vi "ADC Data capture and Process Original - Copy (2).vi"(0 "ADC Output Read Method":T2(ring)=enum."Read .dat file", 1 "Select the Tab to project":T1(ring)=enum."ADC Sine", 2 "ADC Input":enum16{"Sine Wave", "Ramp / Triangle"}(ring), 3 "No.of samples(SNR)":i32=4096, 4 "Resolution":i32=12, 5 "active edge":i32(ring)=10280, 6 "Inputs for Dyanmic para":T9={"Fundamental Frequency"=100000.0, "Sampling Frequncy"=3999610.0, "No of Harmonics"=9, "Window"=enum."7 Term B-Harris", "Blackman (fundamental power) bins)"=1.0}, 7 "Samples per Channel":i32=4096 caption="No.of Samples(capture)", 8 "Oversampling":bool, 9 "Oversampling ratio":i32, 10 "Drop LSB":bool, 11 "Save data":T15, 12 "Waveform":i64[](array[numeric]), 13 "Path to Read":path=path "C/Users/a0230227/Desktop/save.dat", 14 "Start & Stop Bit":cluster{"Start":i32, "Stop":i32}={"Start"=40, "Stop"=4055}, 15 "length":i32=4096, 17 "Set_Freq":dbl=100017.0, 24 "path to save":T14={"Path to Save plot"=path "D/Tenor_176P/DYN_PAR_C004/DAT/D001_TEMPP30C_VDD1.2_VDDA3.3_16B_SE_ADCA__vicA_aggX_PLT_CAP_200821_1740_33.jpg", "Path to Raw Data plot"=path "D/Tenor_176P/DYN_PAR_C004/DAT/D001_TEMPP30C_VDD1.2_VDDA3.3_16B_SE_ADCA__vicA_aggX_RAW_DAT_200821_1740_33.csv"}) -> (18 "Min Max":T4, 19 "detected Throughput":dbl, 20 "output cluster":T7, 21 "Dynamic Parameters":T8, 22 "max code":ext, 23 "min code":ext, 25 "Valid Capture":bool)   [LabVIEW 2019] (continued)
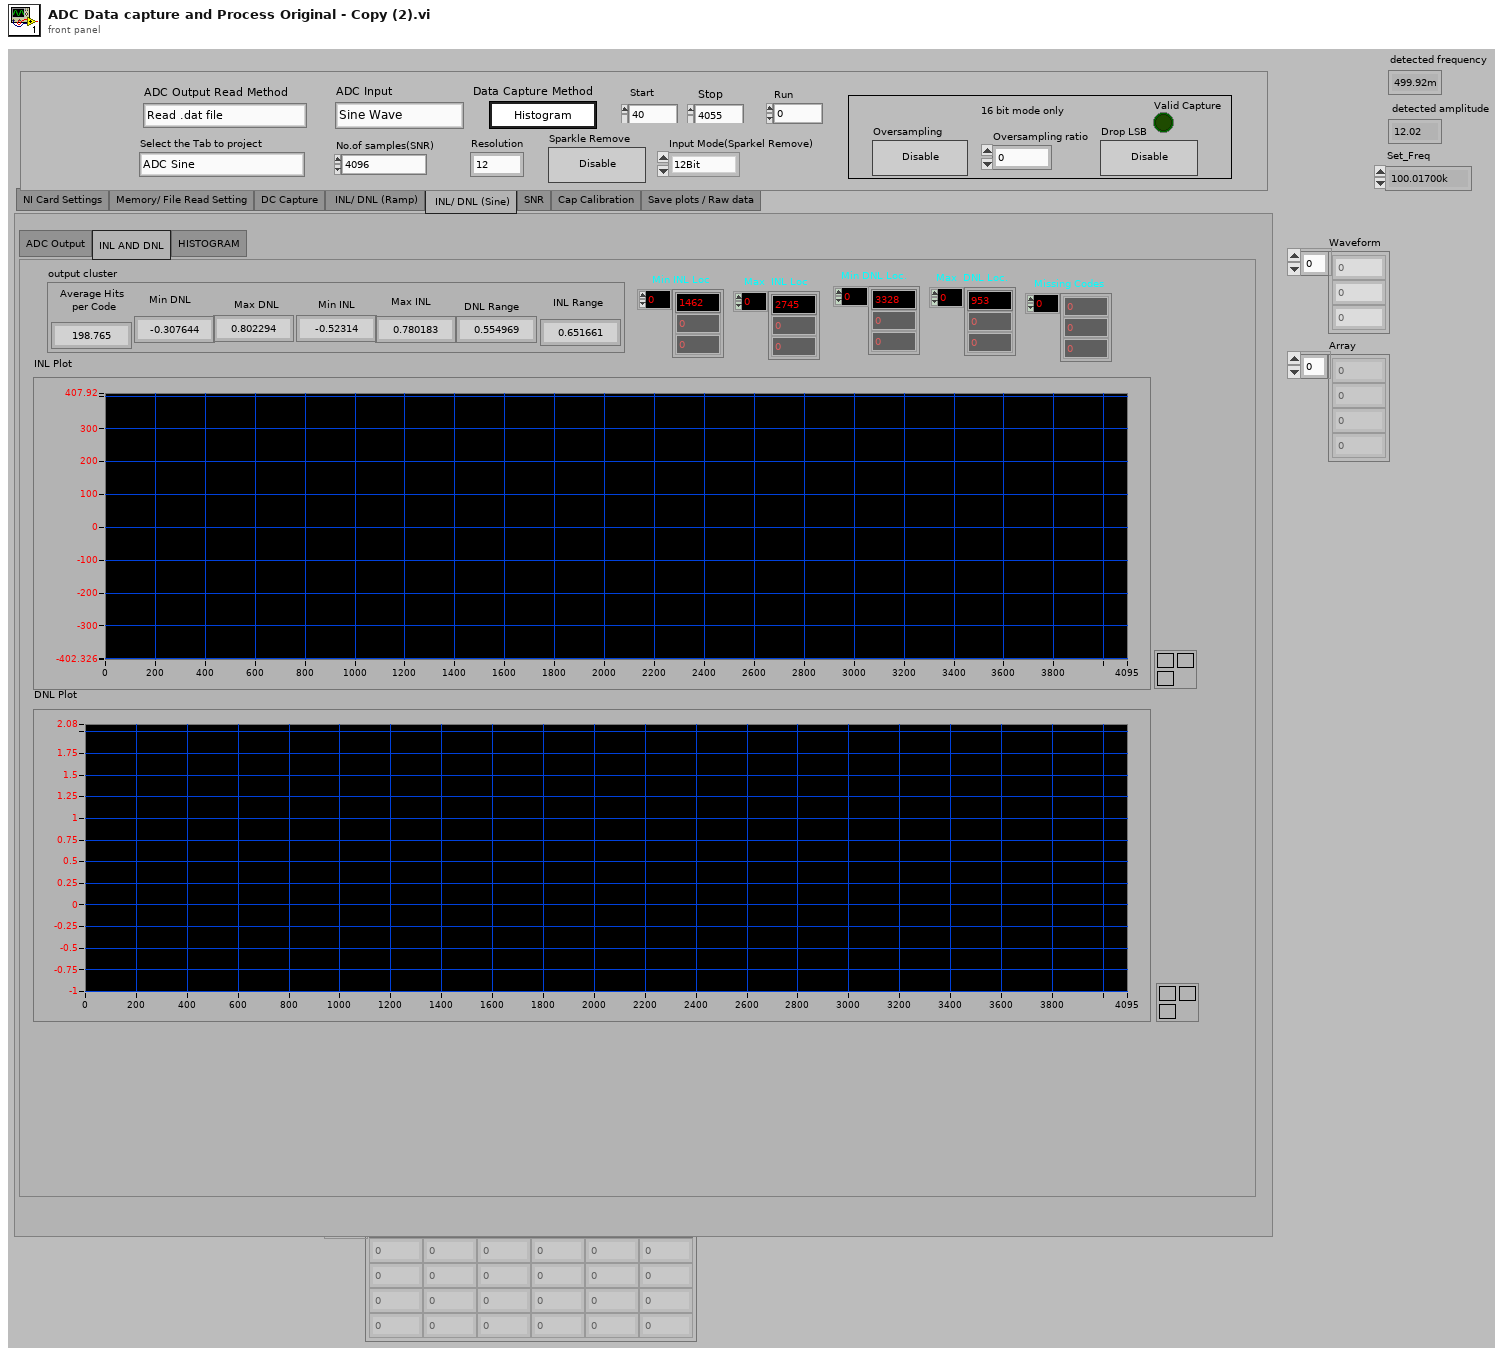
[diagram p1: front panel]
types:
  T1 = enum32{"NI Card Settings", "Memory Read Setting", "DC Capture", "ADC Ramp", "ADC Sine", "SNR", "Cap Calibration"}
  T2 = enum32{"Read from Memory", "Read .dat file", "NI Card Capture", "None"}
  T3 = enum32{"NI Card Settings", "Memory/ File Read Setting", "DC Capture", " INL/ DNL (Ramp)", " INL/ DNL (Sine)", "SNR", "Cap Calibration", "Save plots / Raw data"}
  T4 = cluster{"Min":dbl, "Max":dbl, "delta":dbl, "Average Code":dbl, "Standard Deviation":dbl}
  T5 = cluster{"Min INL":dbl, "Max INL":dbl, "Min DNL":dbl, "Max DNL":dbl, "INL Range":dbl, "DNL Range":dbl, "Avg Hits/Code":dbl}
  T6 = enum32{"ADC Output", "TRIMMED DATA", "INL AND DNL", "HISTOGRAM"}
  T7 = cluster{"Average Hits \nper Code ":dbl, "Min DNL":dbl, "Min INL":dbl, "Max INL":dbl, "Max DNL":dbl, "DNL Range":dbl, "INL Range":dbl}
  T8 = cluster{"SNR":dbl, "SNRD":dbl, "THD":dbl, "ENOB (SNRD)":dbl, "SFDR":dbl, "ENOB (SNR)":dbl, "Noise Power":dbl, "Signal power":dbl}
  T9 = cluster{"Fundamental Frequency":dbl, "Sampling Frequncy":dbl, "No of Harmonics":u8, "Window":enum16{"None ", "Hanning", "Hamming", "Blackman-Harris", "Exact Blackman", "Blackman", "Flat Top", "4 Term B-Harris ", "7 Term B-Harris"}, "Blackman (fundamental power) bins)":dbl}
  T10 = enum32{"ADC Output", "FFT Magnitude plot", " FFT plot"}
  T11 = cluster{"Ideal Power Bin":dbl, "Actual Power Bin":dbl, "Signal Strength (dB)":dbl}
  T12 = cluster{"ADC Reference(V)":dbl, "Bin Width":dbl, "PSRR/ CMRR  ":bool}
  T13 = cluster{"Fundamental Frequnecy (Calculated)":dbl, "Harmonic Frequencies":dbl[], "Harmonic Amplitudes":dbl[]}
  T14 = cluster{"Path to Save plot":path, "Path to Raw Data plot":path}
  T15 = cluster{"Save INL/DNL Plot(Ramp)":bool, "Save SNR Plot":bool, "Save INL/DNL Plot(Sine)":bool, "Save INL/DNL Raw Data(Ramp)":bool, "Save SNR Raw Data":bool, "Save INL/DNL Raw Data(Sine)":bool, "Save DC Raw data":bool, "Save  Raw Data(Sine)":bool}
  T16 = enum16{"Initialize", "Read output", "Post process", "Cap Calib", "Save data", "Exit"}
  T17 = cluster{"Average Hits \nper Code ":dbl, "Min\nDNL":dbl, dbl, dbl, "Max\nDNL":dbl, dbl, dbl}
  T18 = enum16{"None ", "Hanning", "Hamming", "Blackman-Harris", "Exact Blackman", "Blackman", "Flat Top", "4 Term B-Harris ", "7 Term B-Harris"}
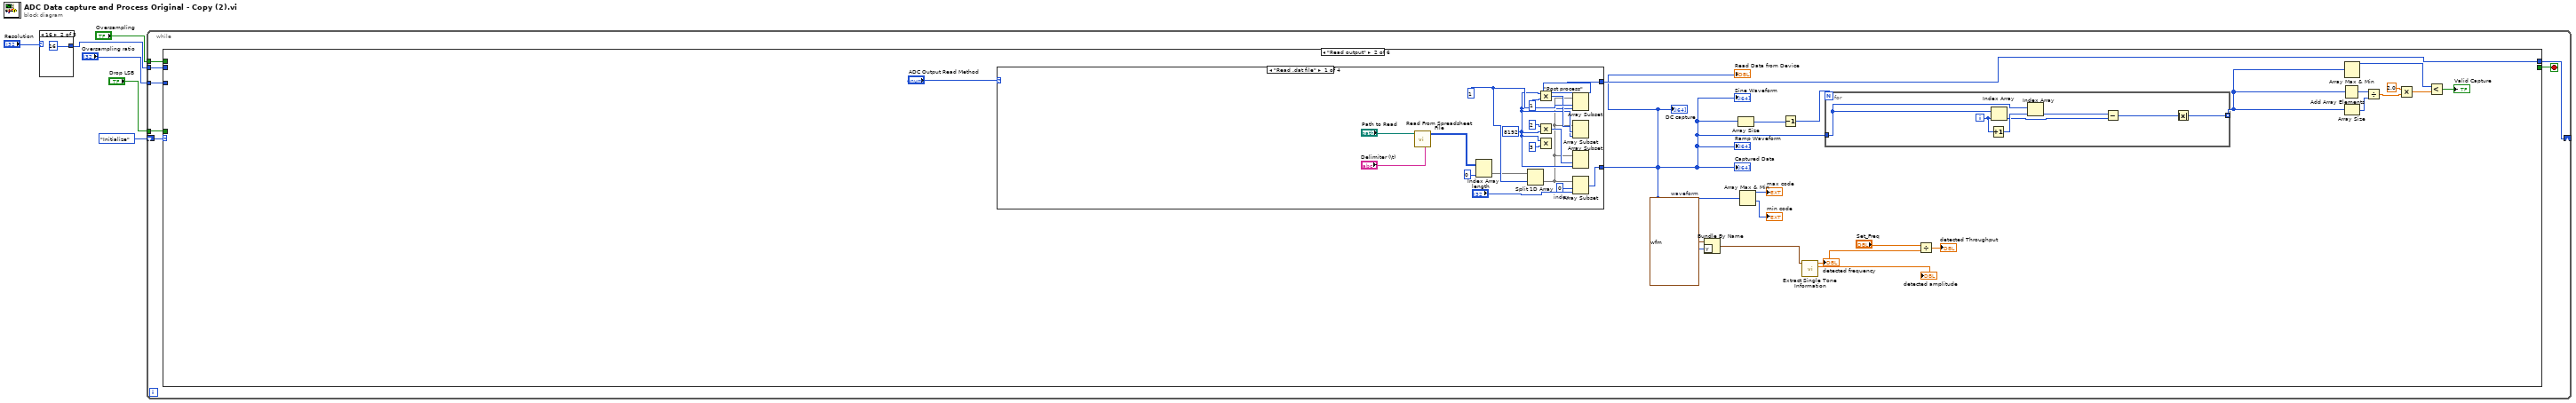
[diagram p0: block diagram]
diagram:
  n1 = case shown="16" "Resolution" {
    tunnel: [18 16 14 12 10] -> w5
    frame 18 {
    }
    frame 16 {
    }
    frame 14, Default {
    }
    frame 12 {
    }
    frame 10 {
    }
  }
  n2 = while {
    shift-right: [w17] -> _
    shift-left: T16."Initialize" -> [w18]
    tunnel: w5 -> [w15]
    tunnel: "Oversampling" -> [w14]
    tunnel: "Drop LSB" -> [w13]
    tunnel: "Oversampling ratio" -> [w12]
    stop <- w16 stop-if-true
    n3 = case shown="\"Read output\"" w18 {
      tunnel: [T16."Read output" w41 w124 T16."Save data" T16."Exit" _] -> w17
      tunnel: [_ _ _ _ _ TRUE] -> w16
      tunnel: w15 -> [_ _ w131 _ _ _]
      tunnel: w14 -> [_ _ w121 _ _ _]
      tunnel: w13 -> [_ _ w123 _ _ _]
      tunnel: w12 -> [_ _ w122 _ _ _]
      frame "Initialize", Default {
        n4 = local read "No.of samples(SNR)"() -> (w19:i32)
        n5 = local write "Samples per Channel"(w19) -> ()
      }
      frame "Read output" {
        w26 = waveform(i64) {"t0"=timestamp(0 s since 1904-01-01), "dt"=1.0, "Y"=[]}  # waveform
        n6 = case shown="\"Read .dat file\"" "ADC Output Read Method" {
          tunnel: [w51 _ w70 "Waveform"] -> w27
          tunnel: [T16."Post process" _ T16."Post process" T16."Post process"] -> w41
          frame "Read .dat file" {
            w50 = 0  # index
            w56 = 8192 ("index")
            w61 = 1 ("index")
            n7 = call-poly <vilib>:"Read From Spreadsheet File.vi"("delimiter (\\t)"="Delimiter (\\t)", "file path (dialog if empty)"="Path to Read") -> ("all rows"=w63:i64[][])  [unwired: 5 in, 4 out]
            n8 = Index Array(array=w63, index (col)=0 ("disabled index (col)")) -> (element=w54:i64[])  [unwired: 1 in]
            n9 = Split 1D Array(array=w54, index=w61) -> (second subarray=w52:i64[])  [unwired: 1 out]
            n10 = Multiply(x=w56, y=1) -> (x*y=w59:i32)
            n11 = Multiply(x=2 ("y"), y=w56) -> (x*y=w57:i32)
            n12 = Multiply(x=w56, y=3) -> ()  [unwired: 1 out]
            n13 = Array Subset(array=w52, index=w61, length=w56) -> ()  [unwired: 1 out]
            n14 = Array Subset(array=w52, index=w59, length=w56) -> ()  [unwired: 1 out]
            n15 = Array Subset(array=w52, index=w57, length=w56) -> ()  [unwired: 1 out]
            n16 = Array Subset(array=w52, index=w50, length="length") -> (w51:i64[])
          }
          frame "None" {
          }
          frame "NI Card Capture", Default {
            n17 = case shown="\"Sine Wave\", Default" "ADC Input" {
              tunnel: "Port" -> [w87 w107]
              tunnel: "Source" -> [w86 w106]
              tunnel: "Rate" -> [w85 w105]
              tunnel: "Timeout" -> [w84 w104]
              tunnel: [_ w102] -> w69
              tunnel: [w80 w103] -> w70
              tunnel: "No.of samples(SNR)" -> [w83 w101]
              tunnel: "Samples per Channel" -> [w81 w100]
              tunnel: "Sparkle Remove" -> [w79 _]
              tunnel: "active edge" -> [w78 w98]
              frame "Sine Wave", Default {
                n18 = disable-structure shown="Disabled" {
                  disable-tunnel: w87 -> [w97 _]
                  disable-tunnel: w86 -> [w96 _]
                  disable-tunnel: w85 -> [w95 _]
                  disable-tunnel: w84 -> [w94 _]
                  disable-tunnel: w83 -> [w93 _]
                  disable-tunnel: FALSE ("Histogram Capture Method SNR") -> [w92 _]
                  disable-tunnel: w81 -> [w91 _]
                  disable-tunnel: [w90 _] -> w80
                  disable-tunnel: w79 -> [w89 _]
                  disable-tunnel: w78 -> [w88 _]
                  frame Disabled {
                    n19 = call "DATA_CAPTURE_SNR.vi"("Port"=w97, "Source"=w96, "No. of samples to process"=w93, "Samples per Channel"=w91, "Rate"=w95, "active edge"=w88, "timeout"=w94, "Histogram Capture Method SNR"=w89, "NI card Cont/Single Capture"=w92) -> ("Waveform"=w90:u32[])  [unwired: 5 in, 5 out]
                  }
                  frame Enabled {
                  }
                }
              }
              frame "Ramp / Triangle" {
                n20 = disable-structure shown="Disabled" {
                  disable-tunnel: w107 -> [w118 _]
                  disable-tunnel: w106 -> [w117 _]
                  disable-tunnel: w105 -> [w116 _]
                  disable-tunnel: w104 -> [w115 _]
                  disable-tunnel: [w114 _] -> w103
                  disable-tunnel: [w113 _] -> w102
                  disable-tunnel: w101 -> [w112 _]
                  disable-tunnel: w100 -> [w110 _]
                  disable-tunnel: FALSE ("Histogram Capture Method SNR") -> [w109 _]
                  disable-tunnel: w98 -> [w108 _]
                  frame Disabled {
                    n21 = call "DATA_CAPTURE_SNR.vi"("Port"=w118, "Source"=w117, "No. of samples to process"=w112, "Samples per Channel"=w110, "Rate"=w116, "active edge"=w108, "timeout"=w115, "Histogram Capture Method SNR"=w109, "NI card Cont/Single Capture"=FALSE ("Histogram Capture Method SNR")) -> ("Waveform"=w114:u32[], "Trimmed Wave"=w113:u32[])  [unwired: 5 in, 4 out]
                  }
                  frame Enabled {
                  }
                }
              }
            }
            "Trimmed Wave" <- w69
          }
          frame "Read from Memory" {
          }
        }
        "Ramp Waveform" <- w27
        "Sine Waveform" <- w27
        "Read Data from Device" <- w27
        "Captured Data" <- w27
        "DC capture" <- w27
        n22 = Bundle By Name(cluster=w26, "Y"=w27) -> (w25:waveform(i64))
        n23 = Array Size(array=w27) -> (size(s)=w37:i32)
        n24 = Array Max & Min(array=w27) -> (max value=→"max code":i64, min value=→"min code":i64)  [unwired: 2 out]
        n25 = Decrement(x=w37) -> (x-1=w36:i32)
        n26 = call-poly <vilib>:"Extract Single Tone Information.vi"("time signal in"=w25) -> ("detected amplitude"=→"detected amplitude":dbl, "detected frequency"=w22:dbl)  [unwired: 5 in, 4 out]
        "detected frequency" <- w22
        n27 = for {
          N: w36 -> [_]
          tunnel: w27 -> [w48]
          tunnel: [w42] -> w34 mode=indexing
          i -> [w46]
          n28 = Increment(x=w46) -> (x+1=w47:i32)
          n29 = Index Array(array=w48, index=w46) -> (element=w44:i64)
          n30 = Index Array(array=w48, index=w47) -> (element=w45:i64)
          n31 = Subtract(x=w45, y=w44) -> (x-y=w43:i64)
          n32 = Absolute Value(x=w43) -> (abs(x)=w42:i64)
        }
        n33 = Divide(x="Set_Freq", y=w22) -> (x/y=→"detected Throughput":dbl)
        n34 = Add Array Elements(numeric array=w34) -> (sum=w32:i64)
        n35 = Array Max & Min(array=w34) -> (max value=w29:i64)  [unwired: 3 out]
        n36 = Array Size(array=w34) -> (size(s)=w31:i32)
        n37 = Divide(x=w32, y=w31) -> (x/y=w33:dbl)
        n38 = Multiply(x=2.0, y=w33) -> (x*y=w28:dbl)
        n39 = Less?(x=w29, y=w28) -> (x < y?=→"Valid Capture":bool)
      }
      frame "Post process" {
        n40 = local read "Select the Tab to project"() -> (w137:T1)
        n41 = local read "Read Data from Device"() -> (w128:dbl[])
        n42 = local read "No.of samples(SNR)"() -> (w130:i32)
        n43 = Equal?(x=w137, y=T1."Cap Calibration" ("Select the Tab to project")) -> (x = y?=w138:bool)
        n44 = Unbundle By Name("Start & Stop Bit") -> ("Start"=w133:i32, "Stop"=w132:i32)
        n45 = Select(t=T1."ADC Sine" ("Select the Tab to project"), s=w138, f=w137) -> (s? t:f=w136:T1)
        n46 = case shown="\"SNR\"" w136 {
          tunnel: w128 -> [w143 w259 w331 w396]
          tunnel: "Data Capture Method" -> [w140 w257 w364 _]
          tunnel: w133 -> [_ w256 w363 _]
          tunnel: w132 -> [_ w255 w362 _]
          tunnel: w131 -> [_ w258 w361 w395]
          tunnel: w130 -> [_ _ _ w397]
          tunnel: [_ w254 w349 _] -> w129
          tunnel: [T16."Save data" T16."Save data" T16."Cap Calib" T16."Save data"] -> w124
          tunnel: w121 -> [_ _ w328 w393]
          tunnel: w123 -> [_ _ w327 w392]
          tunnel: w122 -> [_ _ w329 w391]
          frame "DC Capture", Default {
            n47 = property on="Raw Data CH2" class="Arr (strict)"("Visible"="CH Swtich (To see other CH O/P)") -> ()  [unwired: 2 in, 2 out]
            n48 = property on="Standard Deviation (CH2)" class="DigNum (strict)"("Visible"="CH Swtich (To see other CH O/P)") -> ()  [unwired: 2 in, 2 out]
            n49 = property on="Raw Data CH1" class="Arr (strict)"("Visible"="CH Swtich (To see other CH O/P)") -> ()  [unwired: 2 in, 2 out]
            n50 = property on="Average Code (CH2)" class="DigNum (strict)"("Visible"="CH Swtich (To see other CH O/P)") -> ()  [unwired: 2 in, 2 out]
            n51 = case shown="False" w140 {
              tunnel: w143 -> [w146 w214]
              tunnel: "CH Swtich (To see other CH O/P)" -> [w145 _]
              tunnel: [w144 w200] -> w139
              frame False {
                n52 = case shown="True" w145 {
                  tunnel: w146 -> [w151 w188]
                  tunnel: [w147 w180] -> w144
                  frame True {
                    w157 = 10 ("index")
                    w170 = 10 ("index")
                    n53 = Decimate 1D Array(w151) -> (w167:dbl[], w158:dbl[])
                    "Raw Data CH2" <- w167
                    "Raw Data CH1" <- w158
                    n54 = Split 1D Array(array=w167, index=w170) -> (second subarray=w169:dbl[])  [unwired: 1 out]
                    n55 = Split 1D Array(array=w158, index=w157) -> (second subarray=w166:dbl[])  [unwired: 1 out]
                    n56 = Array Size(array=w169) -> (size(s)=w171:i32)
                    n57 = Array Size(array=w166) -> (size(s)=w165:i32)
                    n58 = Subtract(x=w171, y=w170) -> (x-y=w174:i32)
                    n59 = Subtract(x=w165, y=w157) -> (x-y=w155:i32)
                    n60 = Split 1D Array(array=w169, index=w174) -> (first subarray=w173:dbl[])  [unwired: 1 out]
                    n61 = Split 1D Array(array=w166, index=w155) -> (first subarray=w163:dbl[])  [unwired: 1 out]
                    n62 = Array Size(array=w173) -> (size(s)=w172:i32)
                    n63 = Array Size(array=w163) -> (size(s)=w164:i32)
                    n64 = To Double Precision Float(number=w173) -> (double precision float=w175:dbl[])
                    n65 = To Double Precision Float(number=w163) -> (double precision float=w154:dbl[])
                    n66 = Add Array Elements(numeric array=w175) -> (sum=w179:dbl)
                    n67 = Add Array Elements(numeric array=w154) -> (sum=w159:dbl)
                    n68 = Divide(x=w179, y=w172) -> (x/y=w152:dbl)
                    "Average Code (CH2)" <- w152
                    n69 = Divide(x=w159, y=w164) -> (x/y=w149:dbl)
                    n70 = Subtract(x=w175, y=w152) -> (x-y=w178:dbl[])
                    n71 = Subtract(x=w154, y=w149) -> (x-y=w160:dbl[])
                    n72 = Square(x=w178) -> (x^2=w177:dbl[])
                    n73 = Square(x=w160) -> (x^2=w161:dbl[])
                    n74 = Add Array Elements(numeric array=w177) -> (sum=w176:dbl)
                    n75 = Add Array Elements(numeric array=w161) -> (sum=w162:dbl)
                    n76 = Divide(x=w176, y=w172) -> (x/y=w168:dbl)
                    n77 = Divide(x=w162, y=w164) -> (x/y=w156:dbl)
                    n78 = Square Root(x=w168) -> (sqrt(x)=→"Standard Deviation (CH2)":dbl)
                    n79 = Square Root(x=w156) -> (sqrt(x)=w148:dbl)
                    n80 = local read "Min Max"() -> (w150:T4)
                    n81 = Bundle By Name(cluster=w150, "Average Code"=w149, "Standard Deviation"=w148) -> (w147:T4)
                  }
                  frame False {
                    w192 = 10 ("index")
                    n82 = Split 1D Array(array=w188, index=w192) -> (second subarray=w199:dbl[])  [unwired: 1 out]
                    n83 = Array Size(array=w199) -> (size(s)=w198:i32)
                    n84 = Subtract(x=w198, y=w192) -> (x-y=w190:i32)
                    n85 = Split 1D Array(array=w199, index=w190) -> (first subarray=w187:dbl[])  [unwired: 1 out]
                    n86 = Array Size(array=w187) -> (size(s)=w197:i32)
                    n87 = To Double Precision Float(number=w187) -> (double precision float=w189:dbl[])
                    n88 = Add Array Elements(numeric array=w189) -> (sum=w193:dbl)
                    n89 = Divide(x=w193, y=w197) -> (x/y=w182:dbl)
                    n90 = Subtract(x=w189, y=w182) -> (x-y=w194:dbl[])
                    n91 = Square(x=w194) -> (x^2=w195:dbl[])
                    n92 = Add Array Elements(numeric array=w195) -> (sum=w196:dbl)
                    n93 = Divide(x=w196, y=w197) -> (x/y=w191:dbl)
                    n94 = Array Max & Min(array=w187) -> (max value=w184:dbl, min value=w183:dbl)  [unwired: 2 out]
                    n95 = local read "Min Max"() -> (w186:T4)
                    n96 = Subtract(x=w184, y=w183) -> (x-y=w185:dbl)
                    n97 = Square Root(x=w191) -> (sqrt(x)=w181:dbl)
                    n98 = Bundle By Name(cluster=w186, "Standard Deviation"=w181, "Average Code"=w182, "Max"=w184, "Min"=w183, "delta"=w185) -> (w180:T4)
                  }
                }
              }
              frame True {
                n99 = for {
                  tunnel: w214 -> [w247] mode=indexing
                  shift-right: [w251] -> w223
                  shift-left: 0.0 ("x*y") -> [w252]
                  tunnel: w214 -> [w250]
                  tunnel: [w249] -> w222
                  shift-right: [w238] -> _
                  shift-left: TRUE ("x != 0?") -> [w245]
                  shift-right: [w241] -> w205
                  shift-left: i32[] [] -> [w242]
                  i -> [w244]
                  n100 = Add Array Elements(numeric array=w250) -> (sum=w249:dbl)
                  n101 = Not Equal To 0?(x=w247) -> (x != 0?=w246:bool)
                  n102 = Multiply(x=w247, y=w244) -> (x*y=w248:dbl)
                  n103 = Build Array (concatenate)(w242, w244) -> (w243:i32[])
                  n104 = And(x=w245, y=w246) -> (x .and. y?=w240:bool)
                  n105 = Add(x=w252, y=w248) -> (x+y=w251:dbl)
                  n106 = Select(t=w243, s=w240, f=w242) -> (s? t:f=w241:i32[])
                  n107 = Select(t=FALSE ("x != 0?"), s=w240, f=TRUE ("x != 0?")) -> (s? t:f=w238:bool)
                }
                n108 = Divide(x=w223, y=w222) -> (x/y=w201:dbl)
                n109 = Array Size(array=w205) -> (size(s)=w203:i32)
                n110 = Index Array(array=w205, index=0) -> (element=w206:i32)
                n111 = Split 1D Array(array=w214, index=w206) -> (second subarray=w209:dbl[])  [unwired: 1 out]
                n112 = Subtract(x=w203, y=15 ("x")) -> (x-y=w202:i32)
                n113 = Array Max & Min(array=w209) -> (max index (indices)=w217:i32)  [unwired: 3 out]
                n114 = Greater?(x=w217, y=w202) -> (0:w218:bool)
                n115 = case shown="True" w218 {
                  tunnel: w217 -> [w226 w233]
                  tunnel: [w225 w233] -> w213
                  tunnel: 10 ("y") -> [w230 w232]
                  tunnel: w209 -> [w229 w236]
                  tunnel: [w226 w235] -> w212
                  tunnel: [_ w231] -> w207
                  frame True {
                    n116 = Subtract(x=w226, y=w230) -> (x-y=w227:i32)
                    n117 = Split 1D Array(array=w229, index=w227) -> (first subarray=w228:dbl[])  [unwired: 1 out]
                    n118 = Array Max & Min(array=w228) -> (max index (indices)=w225:i32)  [unwired: 3 out]
                  }
                  frame False {
                    n119 = Add(x=w233, y=w232) -> (x+y=w231:i32)
                    n120 = Split 1D Array(array=w236, index=w231) -> (second subarray=w234:dbl[])  [unwired: 1 out]
                    n121 = Array Max & Min(array=w234) -> (max index (indices)=w235:i32)  [unwired: 3 out]
                  }
                }
                n122 = Add(x=w206, y=w213) -> (x+y=w210:i32)
                n123 = Compound Arithmetic op=ADD(w206, w212, w207) -> (w211:i32)
                n124 = Subtract(x=w211, y=w210) -> (x-y=w216:i32)
                n125 = local read "Min Max"() -> (w221:T4)
                n126 = Bundle By Name(cluster=w221, "Average Code"=w201, "Min"=w210, "Max"=w211, "delta"=w216) -> (w200:T4)
              }
            }
            "Min Max" <- w139
          }
          frame "ADC Ramp" {
            n127 = stacked-sequence {
              seq-local: [w261 _ _] -> [_ w285 _]
              seq-local: [_ w281 _] -> [_ _ w311]
              seq-local: [_ w280 _] -> [_ _ w310]
              seq-local: [_ w279 _] -> [_ _ w299]
              seq-local: [w262 _ _] -> [_ w278 _]
              tunnel: w259 -> [w264 _ _]
              tunnel: w258 -> [w266 _ _]
              tunnel: w257 -> [w265 _ _]
              tunnel: w256 -> [_ w284 _]
              tunnel: w255 -> [_ w283 _]
              tunnel: [w261 _ _] -> w254
              frame #0 {
                n128 = local read "Trimmed Wave"() -> (w260:u32[])
                n129 = Scale By Power Of 2(n=w266, x=ext 1.0) -> (x*2^n=w262:ext)
                n130 = Initialize Array(0 ("element"), w262) -> (w270:i32[])
                n131 = for {
                  shift-right: [w273] -> w263
                  shift-left: w270 -> [w274]
                  tunnel: 0.0 -> [w272]
                  tunnel: w260 -> [w271] mode=indexing
                  n132 = Subtract(x=w271, y=w272) -> (x-y=w275:dbl)
                  n133 = in-place {
                    n134 = in-place-array #1(w274, w275) -> (w277:i32)
                    n135 = Increment(x=w277) -> (x+1=w276:i32)
                    n136 = in-place-array #1(w276) -> (w273:i32[])  [unwired: 1 out]
                  }
                }
                n137 = Select(t=w264, s=w265, f=w263) -> (s? t:f=w261:dbl[])
                "Histogram waveform" <- w261
              }
              frame #1 {
                n138 = Subtract(x=w283, y=w284) -> (x-y=w286:i32)
                n139 = Split 1D Array(array=w285, index=w284) -> (second subarray=w293:dbl[])  [unwired: 1 out]
                n140 = Split 1D Array(array=w293, index=w286) -> (first subarray=w287:dbl[])  [unwired: 1 out]
                n141 = Add Array Elements(numeric array=w287) -> (sum=w290:dbl)
                n142 = Array Size(array=w287) -> (size(s)=w289:i32)
                n143 = Divide(x=w290, y=w289) -> (x/y=w279:dbl)
                n144 = Initialize Array(w279, w278) -> (w288:dbl[])
                n145 = Replace Array Subset(array=w288, new element=w287, index=w284) -> (w292:dbl[])
                n146 = Divide(x=w292, y=w279) -> (x/y=w291:dbl[])
                n147 = Decrement(x=w291) -> (x-1=w281:dbl[])
                "DNL_Ramp" <- w281
                n148 = for {
                  shift-right: [w295] -> _
                  shift-left: 0.0 ("x") -> [w296]
                  tunnel: [w295] -> w280 mode=indexing
                  tunnel: w281 -> [w294] mode=indexing
                  n149 = Add(x=w296, y=w294) -> (x+y=w295:dbl)
                }
                "INL_Ramp" <- w280
              }
              frame #2 {
                n150 = Array Max & Min(array=w311) -> (max value=w302:dbl, min value=w303:dbl)  [unwired: 2 out]
                n151 = Array Max & Min(array=w310) -> (max value=w304:dbl, min value=w305:dbl)  [unwired: 2 out]
                n152 = Subtract(x=w302, y=w303) -> (x-y=w307:dbl)
                n153 = Subtract(x=w304, y=w305) -> (x-y=w308:dbl)
                n154 = local read "Static Parameters (Ramp)"() -> (w298:T5)
                n155 = Divide(x=w307, y=2.0) -> (x/y=w300:dbl)
                n156 = Divide(x=w308, y=2.0) -> (x/y=w301:dbl)
                n157 = disable-structure shown="Enabled" {
                  disable-tunnel: w305 -> [w326 _]
                  disable-tunnel: w304 -> [w325 _]
                  disable-tunnel: w303 -> [w324 _]
                  disable-tunnel: w302 -> [w323 _]
                  disable-tunnel: w301 -> [w314 _]
                  disable-tunnel: w300 -> [w313 _]
                  disable-tunnel: w299 -> [w312 _]
                  frame Disabled {
                    n158 = Increment(x="Run") -> (x+1=w315:dbl)
                    n159 = local write "Run"(w315) -> ()
                    n160 = Build Array(w315, w326, w325, w324, w323, w314, w313, w312) -> (w322:dbl[])
                    n161 = call-poly <vilib>:"Write To Spreadsheet File.vi"("delimiter (\\t)"="," ("delimiter (\\t)"), "transpose? (no:F)"=FALSE, "format (%.3f)"="%.4f", "append to file? (new file:F)"=TRUE, "1D data"=w322, "file path (dialog if empty)"=path "D:/FALCON/ADC/Raw_Data/runtorun.csv") -> ()  [unwired: 2 in, 1 out]
                  }
                  frame Enabled {
                  }
                }
                n162 = Bundle By Name(cluster=w298, "Max INL"=w304, "Min INL"=w305, "Max DNL"=w302, "Min DNL"=w303, "INL Range"=w301, "DNL Range"=w300, "Avg Hits/Code"=w299) -> (→"Static Parameters (Ramp)":T5)
              }
            }
          }
          frame "ADC Sine" {
            n163 = case shown="True" w328 {
              tunnel: w331 -> [w366 w374]
              tunnel: [w367 w372] -> w330
              tunnel: w329 -> [_ w373]
              tunnel: w327 -> [w365 _]
              frame False {
                n164 = case shown="True" w365 {
                  tunnel: w366 -> [w368 w370]
                  tunnel: [w368 w369] -> w367
                  frame False {
                  }
                  frame True {
                    n165 = Divide(x=w370, y=2.0) -> (x/y=w369:dbl[])
                  }
                }
              }
              frame True {
                n166 = Array Size(array=w374) -> (size(s)=w376:i32)
                n167 = Divide(x=w376, y=w373) -> (x/y=w375:dbl)
                n168 = for {
                  N: w375 -> [_]
                  tunnel: w374 -> [w383]
                  tunnel: w373 -> [w378]
                  tunnel: [w377] -> w372 mode=indexing
                  i -> [w382]
                  n169 = Multiply(x=w378, y=w382) -> (x*y=w381:i32)
                  n170 = Array Subset(array=w383, index=w381, length=w378) -> (w380:dbl[])
                  n171 = Add Array Elements(numeric array=w380) -> (sum=w379:dbl)
                  n172 = Divide(x=w379, y=w378) -> (x/y=w377:dbl)
                }
              }
            }
            n173 = call "Sinewave_Linearity_trial_F027.vi"("Array"=w330, "Histogram Capture Method"=w364, "L code"=w363, "UCode"=w362, "Resolution"=w361, "Histogram: h(x)"=w330) -> ("Average Hits \nper Code"=w339:dbl, "Max\nDNL"=w335:dbl, "Min\nDNL"=w338:dbl, "Missing Codes"=→"Missing Codes":i32[], "Max  DNL Loc."=→"Max  DNL Loc.":i32[], "Min DNL Loc."=→"Min DNL Loc.":i32[], "Max  INL Loc"=→"Max  INL Loc":i32[], "Min INL Loc"=→"Min INL Loc":i32[], "Histogram Plot"=w351:dbl[][], "DNL Plot"=w347:dbl[], "INL Plot"=w340:dbl[])  [unwired: 1 in, 2 out]
            "Histogram Plot" <- w351
            "DNL Plot" <- w347
            "INL Plot" <- w340
            n174 = for {
              tunnel: w347 -> [w390] mode=indexing
              tunnel: [w386] -> w346 mode=indexing
              shift-right: [w385] -> _
              shift-left: 16384 ("f") -> [w384]
              i -> [w387]
              n175 = Increment(x=w384) -> (x+1=w385:i32)
              n176 = Greater?(x=w390, y=0.9) -> (0:w388:bool)
              n177 = Select(t=w387, s=w388, f=w384) -> (s? t:f=w386:i32)
            }
            n178 = Subtract(x=w335, y=w338) -> (x-y=w358:dbl)
            n179 = Array Max & Min(array=w340) -> (max value=w336:dbl, min value=w337:dbl)  [unwired: 2 out]
            n180 = Index Array(array=w351, index (col)=1 ("disabled index (col)")) -> (element=w349:dbl[])  [unwired: 1 in]
            n181 = Subtract(x=w336, y=w337) -> (x-y=w360:dbl)
            n182 = Divide(x=w358, y=2.0) -> (x/y=w334:dbl)
            n183 = Divide(x=w360, y=2.0) -> (x/y=w333:dbl)
            n184 = Bundle("Average Hits \nper Code"=w339, "Min\nDNL"=w338, w337, w336, "Max\nDNL"=w335, w334, w333) -> (→"output cluster":T17)  [unwired: 1 in]
            n185 = Sort 1D Array(array=w346) -> (sorted array=w342:i32[])
            n186 = Search 1D Array(1D array=w342, element=16384) -> (index of element=w343:i32)  [unwired: 1 in]
            n187 = Array Subset(array=w342, length=w343) -> (→"Array":i32[])  [unwired: 1 in]
          }
          frame "SNR" {
            n188 = stacked-sequence {
              seq-local: [w418 _ _] -> [_ w479 _]
              seq-local: [w417 _ _] -> [_ _ w504]
              seq-local: [w411 _ _] -> [_ _ w507]
              seq-local: [w410 _ _] -> [_ _ w503]
              seq-local: [w409 _ _] -> [_ _ w502]
              tunnel: w397 -> [w430 _ w505]
              tunnel: w396 -> [w412 _ _]
              tunnel: w395 -> [w414 _ _]
              tunnel: w393 -> [w401 _ _]
              tunnel: w392 -> [w400 _ _]
              tunnel: w391 -> [w399 _ _]
              frame #0 {
                n189 = Unbundle By Name("PSRR/CMRR Input") -> ("ADC Reference(V)"=w413:dbl, "PSRR/ CMRR"=w409:bool)
                n190 = case shown="True" w409 {
                  tunnel: 1.0 ("x") -> [_ w465]
                  tunnel: w414 -> [_ w464]
                  tunnel: w413 -> [_ w462]
                  tunnel: w412 -> [w458 w460]
                  tunnel: [w458 w459] -> w403
                  frame False {
                  }
                  frame True {
                    n191 = Scale By Power Of 2(n=w464, x=w465) -> (x*2^n=w463:dbl)
                    n192 = Divide(x=w462, y=w463) -> (x/y=w461:dbl)
                    n193 = Multiply(x=w460, y=w461) -> (x*y=w459:dbl[])
                  }
                }
                n194 = case shown="True" w401 {
                  tunnel: w403 -> [w440 w448]
                  tunnel: [w441 w446] -> w402
                  tunnel: w399 -> [_ w447]
                  tunnel: w400 -> [w439 _]
                  frame False {
                    n195 = case shown="True" w439 {
                      tunnel: w440 -> [w442 w444]
                      tunnel: [w442 w443] -> w441
                      frame False {
                      }
                      frame True {
                        n196 = Divide(x=w444, y=2.0) -> (x/y=w443:dbl[])
                      }
                    }
                  }
                  frame True {
                    n197 = Array Size(array=w448) -> (size(s)=w450:i32)
                    n198 = Divide(x=w450, y=w447) -> (x/y=w449:dbl)
                    n199 = for {
                      N: w449 -> [_]
                      tunnel: w448 -> [w457]
                      tunnel: w447 -> [w452]
                      tunnel: [w451] -> w446 mode=indexing
                      i -> [w456]
                      n200 = Multiply(x=w452, y=w456) -> (x*y=w455:i32)
                      n201 = Array Subset(array=w457, index=w455, length=w452) -> (w454:dbl[])
                      n202 = Add Array Elements(numeric array=w454) -> (sum=w453:dbl)
                      n203 = Divide(x=w453, y=w452) -> (x/y=w451:dbl)
                    }
                  }
                }
                n204 = Unbundle By Name("Inputs for Dyanmic para") -> ("Window"=w428:T18, "Sampling Frequncy"=w417:dbl, "Fundamental Frequency"=w411:dbl, "No of Harmonics"=w418:u8, "Blackman (fundamental power) bins)"=w427:dbl)
                n205 = Reciprocal(x=w417) -> (1/x=w432:dbl)
                n206 = call-poly <vilib>:"Scaled Time Domain Window.vi"("window"=w428, "X"=w402) -> ("Windowed X"=w436:dbl[])  [unwired: 7 in, 2 out]
                n207 = local read "Dynamic Parameters"() -> (w426:T8)
                n208 = call <vilib>:"Auto Power Spectrum.vi"("dt"=w432, "Signal (V)"=w436) -> ("Power Spectrum (V^2 rms)"=w431:dbl[])  [unwired: 1 out]
                n209 = Logarithm Base 10(1:w431) -> (0:w438:dbl[])
                n210 = call "Calculate_SNR_THD.vi"("Auto Power Spectrum"=w431, "frame size"=w430, "# harmonics"=w418, "window"=w428, "sampling rate"=w417, "fundamental frequency"=w411, "Blackman\n (fundamental power bins)"=w427) -> ("% THD"=w425:dbl, "ENOB(SNRD)"=w420:dbl, "% THD + Noise"=w398:dbl, "ENOB(SNR)"=w421:dbl, "Noise Power"=w424:dbl, "Fundamental frequency Calculated"=w406:dbl, "SNR"=w423:dbl, "Signal power"=w422:dbl, "Harmonic Amplitudes"=w433:dbl[], "Harmonic Frequencies"=w408:dbl[])  [unwired: 3 in]
                n211 = Bundle By Name(cluster=w426, "THD"=w425, "SNRD"=w398, "Noise Power"=w424, "SNR"=w423, "Signal power"=w422, "ENOB (SNR)"=w421, "ENOB (SNRD)"=w420) -> (→"Dynamic Parameters":T8)
                n212 = Logarithm Base 10(1:w433) -> (0:w435:dbl[])
                n213 = Multiply(x=10.0, y=w438) -> (x*y=w410:dbl[])
                "FFT Magnitude Plot (dB)" <- w410
                n214 = local read "Harmonic Details"() -> (w404:T13)
                n215 = Multiply(x=20, y=w435) -> (x*y=w407:dbl[])
                n216 = Bundle By Name(cluster=w404, "Fundamental Frequnecy (Calculated)"=w406, "Harmonic Frequencies"=w408, "Harmonic Amplitudes"=w407) -> (→"Harmonic Details":T13)
              }
              frame #1 {
                n217 = local read "Harmonic Details"() -> (w467:T13)
                n218 = Unbundle By Name(w467) -> ("Harmonic Amplitudes"=w466:dbl[])
                n219 = Decrement(x=w479) -> (x-1=w485:u8)
                n220 = Index Array(array=w466, index=0) -> (element=w481:dbl)
                n221 = Array Subset(array=w466, index=1, length=w485) -> (w483:dbl[])
                n222 = Array Max & Min(array=w483) -> (max value=w480:dbl)  [unwired: 3 out]
                n223 = local read "Dynamic Parameters"() -> (w478:T8)
                n224 = Subtract(x=w481, y=w480) -> (x-y=w477:dbl)
                n225 = Bundle By Name(cluster=w478, "SFDR"=w477) -> (w476:T8)
                n226 = local write "Dynamic Parameters"(w476) -> ()
                n227 = Unbundle By Name(w476) -> ("SNR"=w475:dbl, "SNRD"=w474:dbl, "THD"=w473:dbl, "SFDR"=w472:dbl, "ENOB (SNR)"=w471:dbl, "ENOB (SNRD)"=w470:dbl, "Noise Power"=w469:dbl, "Signal power"=w468:dbl)
                n228 = disable-structure shown="Enabled" {
                  disable-tunnel: w475 -> [w501 _]
                  disable-tunnel: w474 -> [w500 _]
                  disable-tunnel: w470 -> [w488 _]
                  disable-tunnel: w473 -> [w491 _]
                  disable-tunnel: w472 -> [w490 _]
                  disable-tunnel: w471 -> [w489 _]
                  disable-tunnel: w469 -> [w487 _]
                  disable-tunnel: w468 -> [w486 _]
                  frame Disabled {
                    n229 = local read "Run"() -> (w492:dbl)
                    n230 = Increment(x=w492) -> (x+1=w493:dbl)
                    n231 = local write "Run"(w493) -> ()
                    n232 = Build Array(w493, w501, w500, w491, w490, w489, w488, w487, w486) -> (w499:dbl[])
                    n233 = call-poly <vilib>:"Write To Spreadsheet File.vi"("delimiter (\\t)"="," ("delimiter (\\t)"), "transpose? (no:F)"=FALSE, "format (%.3f)"="%.4f", "append to file? (new file:F)"=TRUE, "1D data"=w499, "file path (dialog if empty)"=path "D:/FALCON/ADC/Raw_Data/runtorun.csv") -> ()  [unwired: 2 in, 1 out]
                  }
                  frame Enabled {
                  }
                }
              }
              frame #2 {
                n234 = local read "FFT Magnitude Plot (dB)"() -> (w514:dbl[])
                n235 = Array Size(array=w514) -> (size(s)=w513:i32)
                n236 = Divide(x=w504, y=2.0) -> (x/y=w511:dbl)
                n237 = for {
                  N: w513 -> [_]
                  tunnel: w514 -> [w557]
                  tunnel: [w552] -> w509 mode=indexing
                  tunnel: w513 -> [w555]
                  tunnel: w511 -> [w553]
                  tunnel: [w551] -> w510 mode=indexing
                  tunnel: [w551] -> w506
                  i -> [w556]
                  n238 = Divide(x=w556, y=w555) -> (x/y=w554:dbl)
                  n239 = Index Array(array=w557, index=w556) -> (element=w552:dbl)
                  n240 = Multiply(x=w554, y=w553) -> (x*y=w551:dbl)
                }
                n241 = case shown="True" w502 {
                  tunnel: w507 -> [_ w518]
                  tunnel: w506 -> [_ w519]
                  tunnel: w505 -> [_ w533]
                  tunnel: w504 -> [_ w521]
                  tunnel: w503 -> [_ w525]
                  frame False {
                  }
                  frame True {
                    n242 = Greater?(x=w518, y=w519) -> (0:w520:bool)
                    n243 = case shown="True" w520 {
                      tunnel: [w536 w537] -> w517
                      tunnel: w518 -> [w536 w543]
                      tunnel: w521 -> [_ w542]
                      tunnel: w519 -> [_ _]
                      tunnel: w518 -> [_ w541]
                      frame False {
                      }
                      frame True {
                        n244 = while {
                          tunnel: w542 -> [w550]
                          tunnel: w543 -> [w547]
                          shift-right: [w545] -> _
                          shift-left: w542 -> [w544]
                          shift-left: w542 -> [_]
                          tunnel: [w544] -> w540
                          i -> [w548]
                          stop <- w546 continue-if-true
                          n245 = Increment(x=w548) -> (x+1=w549:i32)
                          n246 = Multiply(x=w550, y=w549) -> (x*y=w545:dbl)
                          n247 = Greater?(x=w547, y=w545) -> (0:w546:bool)
                        }
                        n248 = Subtract(x=w540, y=w541) -> (x-y=w538:dbl)
                        n249 = Sign(1:w538) -> (0:w539:dbl)
                        n250 = Multiply(x=w538, y=w539) -> (x*y=w537:dbl)
                      }
                    }
                    n251 = Multiply(x=w533, y=w517) -> (x*y=w535:dbl)
                    n252 = local read "PSRR/CMRR Input"() -> (w531:T12)
                    n253 = Divide(x=w535, y=w521) -> (x/y=w534:dbl)
                    n254 = Unbundle By Name(w531) -> ("Bin Width"=w516:dbl)
                    n255 = To Long Integer(number=w534) -> (32bit integer=w530:i32)
                    n256 = Subtract(x=w530, y=w516) -> (x-y=w526:dbl)
                    n257 = Add(x=w530, y=w516) -> (x+y=w515:dbl)
                    n258 = Split 1D Array(array=w525, index=w515) -> (first subarray=w529:dbl[])  [unwired: 1 out]
                    n259 = Split 1D Array(array=w529, index=w526) -> (second subarray=w528:dbl[])  [unwired: 1 out]
                    n260 = Array Max & Min(array=w528) -> (max value=w524:dbl, max index (indices)=w527:i32)  [unwired: 2 out]
                    n261 = local read "PSRR/CMRR Output"() -> (w532:T11)
                    n262 = Add(x=w527, y=w526) -> (x+y=w523:dbl)
                    n263 = Bundle By Name(cluster=w532, "Ideal Power Bin"=w530, "Actual Power Bin"=w523, "Signal Strength (dB)"=w524) -> (→"PSRR/CMRR Output":T11)
                  }
                }
                n264 = Bundle(w510, w509) -> (→"FFT Plot":cluster{dbl[], dbl[]})  [unwired: 1 in]
              }
            }
          }
        }
        n265 = Build Array(w128, w129) -> (→"Raw_Histo":dbl[][])
      }
      frame "Cap Calib" {
        n266 = case shown="\"64\"" "Average Window" {
          tunnel: [8 16 32 64] -> w558
          frame "8", Default {
          }
          frame "16" {
          }
          frame "32" {
          }
          frame "64" {
          }
        }
        n267 = case shown="True" "Cap Calibration" {
          tunnel: w558 -> [_ w566]
          frame False {
          }
          frame True {
            n268 = local read "DNL Plot"() -> (w567:dbl[])
            n269 = local read "INL Plot"() -> (w568:dbl[])
            n270 = disable-structure shown="Disabled" {
              disable-tunnel: "INL/DNL Values" -> [w587 _]
              disable-tunnel: "File path (DNL & INL)" -> [w586 _]
              disable-tunnel: "Select Channel" -> [w585 _]
              disable-tunnel: [w584 _] -> w573
              disable-tunnel: [w583 _] -> w572
              disable-tunnel: [w582 _] -> w571
              disable-tunnel: [w581 _] -> w570
              disable-tunnel: [w580 _] -> w569
              disable-tunnel: w568 -> [w579 _]
              disable-tunnel: w567 -> [w578 _]
              disable-tunnel: w566 -> [w577 _]
              frame Disabled {
                n271 = call "Cap_Calibration.vi"("INL"=w579, "DNL"=w578, "From File/ Waveform"=w587, "Select Channel"=w585, "Average Window"=w577, "File path (DNL & INL)"=w586) -> ("ADC TEST 7"=w580:string, "ADC TEST 6"=w581:string, "ADC TEST 5"=w582:string, "Trim Coeff (Binary)"=w584:string[], "Trim Coeff (Integer)"=w583:dbl[])  [unwired: 1 in]
              }
              frame Enabled {
              }
            }
            "Trim Coeff (Binary)" <- w573
            "Trim Coeff (Integer)" <- w572
            "ADC TEST 5" <- w571
            "ADC TEST 6" <- w570
            "ADC TEST 7" <- w569
          }
        }
      }
      frame "Save data" {
        n272 = Unbundle By Name("path to save") -> ("Path to Save plot"=w588:path, "Path to Raw Data plot"=w591:path)
        n273 = disable-structure shown="Enabled" {
          disable-tunnel: w591 -> [w612 w724]
          disable-tunnel: [w604 w724] -> w589
          frame Disabled {
            w602 = "16Hits_Run" ("regular expression")
            n274 = local read "Run"() -> (w603:dbl)
            n275 = Increment(x=w603) -> (x+1=w607:dbl)
            n276 = local write "Run"(w607) -> ()
            n277 = Path To String(path=w612) -> (string=w611:string)
            n278 = Number To Decimal String(number=w607) -> (decimal integer string=w608:string)  [unwired: 1 in]
            n279 = xnode "Match Regular Expression"("input string"=w611, "regular expression"=w602) -> ("before match"=w610:string, "after match"=w609:string)  [unwired: 4 in, 3 out]
            n280 = Concatenate Strings(w602, w608) -> (w606:string)
            n281 = Concatenate Strings(w610, w606, w609) -> (w605:string)
            n282 = String To Path(string=w605) -> (path=w604:path)
          }
          frame Enabled {
          }
        }
        n283 = Unbundle By Name("Save data") -> ("Save INL/DNL Plot(Ramp)"=w598:bool, "Save INL/DNL Raw Data(Ramp)"=w597:bool, "Save INL/DNL Plot(Sine)"=w596:bool, "Save INL/DNL Raw Data(Sine)"=w595:bool, "Save SNR Plot"=w594:bool, "Save SNR Raw Data"=w593:bool, "Save DC Raw data"=w590:bool)  [unwired: 1 out]
        n284 = case shown="\"ADC Ramp\"" "Select the Tab to project" {
          tunnel: w588 -> [w728 w748 w772 _ _]
          tunnel: w589 -> [w729 w749 w771 _ w788]
          tunnel: w598 -> [w726 _ _ _ _]
          tunnel: w597 -> [w725 _ _ _ _]
          tunnel: w596 -> [_ w746 _ _ _]
          tunnel: w595 -> [_ w745 _ _ _]
          tunnel: w594 -> [_ _ w769 _ _]
          tunnel: w593 -> [_ _ w768 _ _]
          tunnel: w590 -> [_ _ _ _ w787]
          frame "ADC Ramp" {
            n285 = case shown="True" w726 {
              tunnel: w728 -> [_ w731]
              frame False {
              }
              frame True {
                n286 = Current VI's Path() -> (path=w732:path)
                n287 = call "Take fron panel screenshot.vi"("VI path"=w732, "Image path"=w731, "Visible area only? (f)"=FALSE, "File type (.jpg)"=enum16{".bmp", ".png", ".jpg"}.".png") -> ()  [unwired: 4 in, 1 out]
              }
            }
            n288 = case shown="True" w725 {
              tunnel: w729 -> [_ w738]
              frame False {
              }
              frame True {
                w737 = "" ("delimiter (\\t)")
